vi "Add Record Call to BD.vi"(8 "error in (no error)":errorcluster, 10 "map":map{string, refnum<vi>}(c390), 11 "VI in":refnum<vi>) -> (0 "error out":errorcluster, 3 "VI out":refnum<vi>)   [LabVIEW 2020, in "Pure Mock Class Generator.lvclass"]
uses:
  Pure Mock Class Generator.lvclass
  <vilib>/Utility/miscctls.llb/LVPointTypeDef.ctl
  Templates/Template VI.vi
  Templates/Templates.lvlib
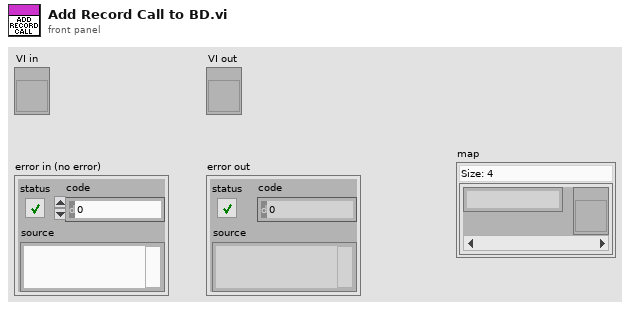
[diagram p1: front panel]
types:
  T1 = typedef "LVPointTypeDef.ctl" = cluster{"Horizontal":i16, "Vertical":i16}
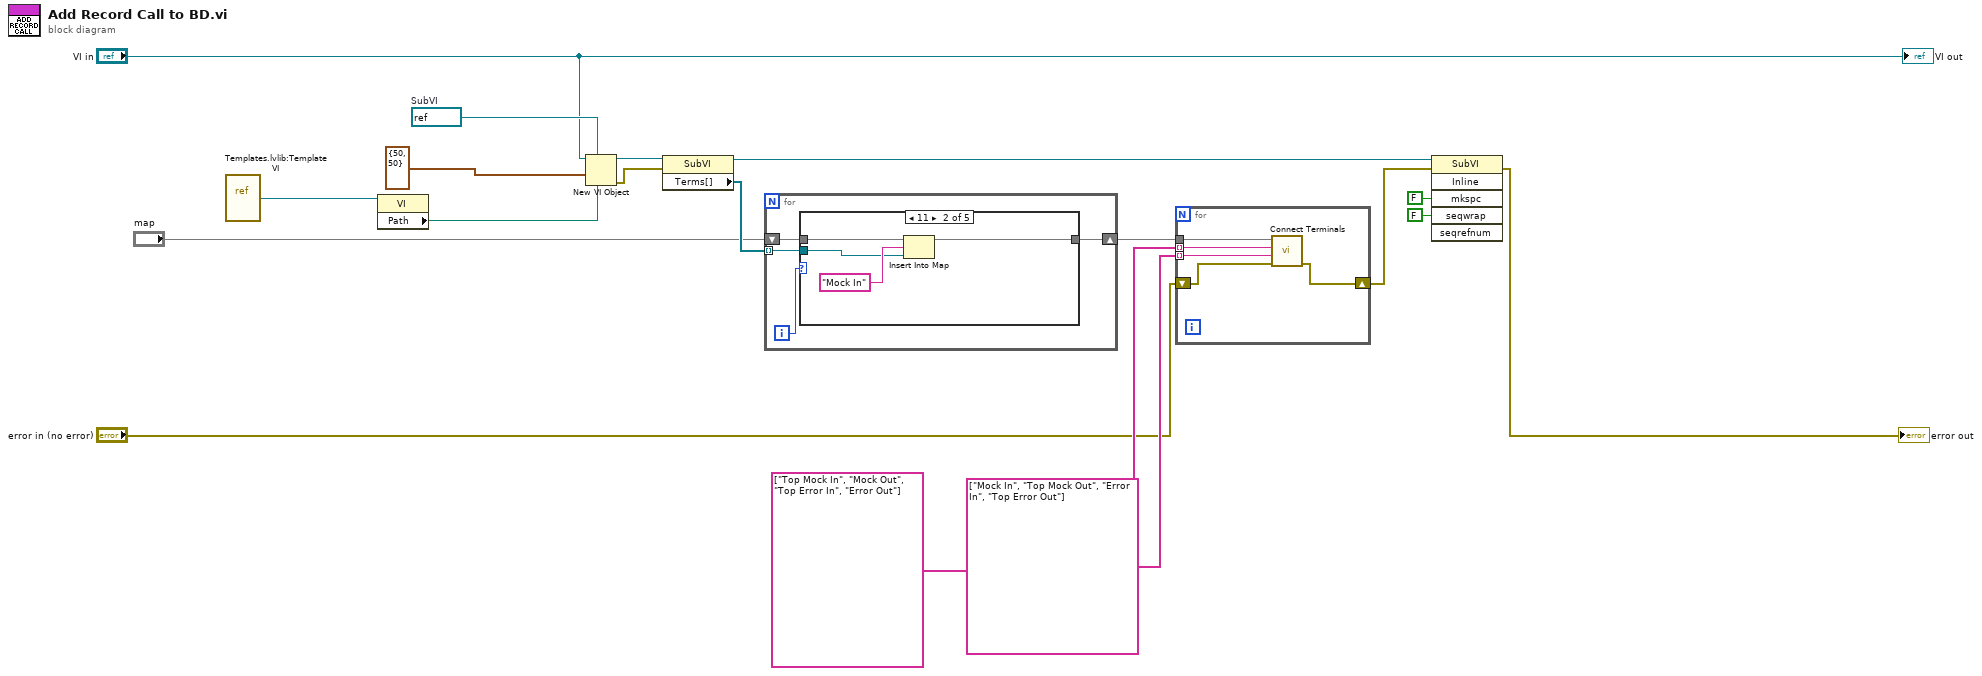
[diagram p0: block diagram]
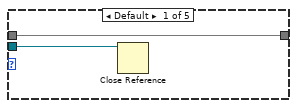
[diagram p2: hidden frame]
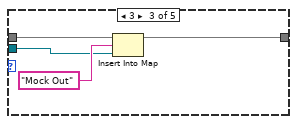
[diagram p3: hidden frame]
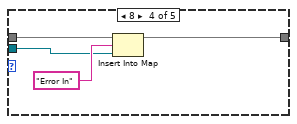
[diagram p4: hidden frame]
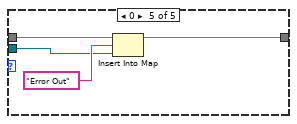
[diagram p5: hidden frame]
diagram:
  w18 = refnum<vi> refnum  # SubVI
  n1 = vi-ref "Templates.lvlib:Template VI.vi"() -> (w16:refnum<vi>)
  n2 = property class="VI"(reference=w16) -> ("Path"=w15:path)  [unwired: 1 in, 2 out]
  n3 = New VI Object(vi object class=w18, owner refnum="VI in", position/next to=T1 {"Horizontal"=50, "Vertical"=50} ("location"), 6:w15) -> (object refnum=w10:refnum<vi>, 0:w13:errorcluster)  [unwired: 4 in]
  n4 = property class="SubVI"(reference=w10, error in=w13) -> (reference out=w9:refnum<vi>, "Terms[]"=w8:refnum<vi>[])  [unwired: 1 out]
  n5 = for {
    tunnel: w8 -> [w21] mode=indexing
    shift-right: [w19] -> w6
    shift-left: "map" -> [w20]
    i -> [w22]
    n6 = case shown="11" w22 {
      tunnel: w21 -> [w24 w26 w30 w34 w38]
      tunnel: w20 -> [w23 w27 w31 w35 w39]
      tunnel: [w23 w25 w29 w33 w37] -> w19
      frame Default {
        n7 = Close Reference(reference=w24) -> ()  [unwired: 1 in, 1 out]
      }
      frame 11 {
        n8 = Insert Into Map(map in=w27, key="Mock In", value=w26) -> (map out=w25:map{string, refnum<vi>})  [unwired: 2 out]
      }
      frame 3 {
        n9 = Insert Into Map(map in=w31, key="Mock Out", value=w30) -> (map out=w29:map{string, refnum<vi>})  [unwired: 2 out]
      }
      frame 8 {
        n10 = Insert Into Map(map in=w35, key="Error In", value=w34) -> (map out=w33:map{string, refnum<vi>})  [unwired: 2 out]
      }
      frame 0 {
        n11 = Insert Into Map(map in=w39, key="Error Out", value=w38) -> (map out=w37:map{string, refnum<vi>})  [unwired: 2 out]
      }
    }
  }
  n12 = for {
    tunnel: w6 -> [w45]
    tunnel: string[] ["Top Mock In", "Mock Out", "Top Error In", "Error Out"] ("Source") -> [w44] mode=indexing
    tunnel: string[] ["Mock In", "Top Mock Out", "Error In", "Top Error Out"] ("Sink") -> [w43] mode=indexing
    shift-right: [w42] -> w3
    shift-left: "error in (no error)" -> [w41]
    n13 = call "Connect Terminals.vi"("error in (no error)"=w41, "Sink"=w43, "Source"=w44, "map"=w45) -> ("error out"=w42:errorcluster)  [unwired: 7 in]
  }
  n14 = invoke class="SubVI" method="Inline"(reference=w9, error in=w3, "mkspc"=FALSE ("Make Space in Block Diagram"), "seqwrap"=FALSE ("Wrap in Sequence")) -> (error out=→"error out":errorcluster)  [unwired: 2 in, 5 out]
  "VI out" <- "VI in"
